vi "SCCSup Build Backend VI Path.vi"(6 "scc operation":T1, 9 "provider location":string, 11 "caller path":path) -> (2 "scc backend VI path":path)   [LabVIEW 2020]
uses:
  <vilib>/SourceControl/sccapi/SCCAPI SCC Operations.ctl
  <vilib>/SourceControl/sccapi/NI_SCC.lvlib
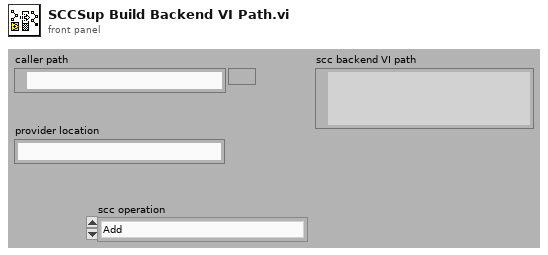
[diagram p1: front panel]
types:
  T1 = typedef "NI_SCC.lvlib/SCCAPI SCC Operations.ctl" = enum16{"Add", "Check In", "Check Out", "Close Project", "Compare Files", "Compare VIs", "Configure Project", "File History", "File Properties", "File Status", "Find All Providers", "Get Advanced Command Options", "Get File Copy", "Get Latest Version", "Get Project Name", "Get StaticVI Path", "Initialize", "Not A Source Control Reference", "Open Project", "Provider Supports Functionality", "Remove", "Run Provider", "Undo Check Out", "Uninitialize", "Is File In Local Path"}
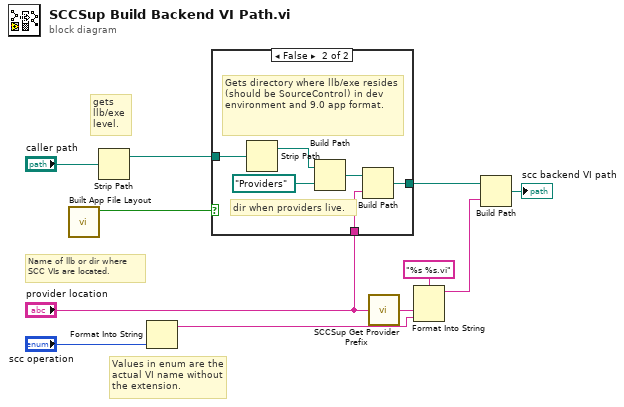
[diagram p0: block diagram]
diagram:
  # "Values in enum are the actual VI name without the extension."
  # "Name of llb or dir where SCC VIs are located."
  # "gets llb/exe level."
  n1 = call <vilib>:"Built App File Layout.vi"() -> ("Legacy Layout?"=w1:bool)  [unwired: 1 in, 10 out]
  n2 = Strip Path(path="caller path") -> (stripped path=w2:path)  [unwired: 1 out]
  n3 = Format Into String("scc operation") -> (resulting string=w3:string)  [unwired: 3 in, 1 out]
  n4 = case shown="False" w1 {
    tunnel: "provider location" -> [_ w18]
    tunnel: w2 -> [w12 w14]
    tunnel: [w12 w16] -> w7
    frame True {
      # "All files are at the same level in an exe, so there is no need to build up a directory heirarchy."
    }
    frame False {
      # "dir when providers live."
      # "Gets directory where llb/exe resides (should be SourceControl) in dev environment and 9.0 app format."
      n5 = Strip Path(path=w14) -> (stripped path=w13:path)  [unwired: 1 out]
      n6 = Build Path(base path=w13, name or relative path=path "Providers") -> (appended path=w17:path)
      n7 = Build Path(base path=w17, name or relative path=w18) -> (appended path=w16:path)
    }
  }
  n8 = call <vilib>:"SCCSup Get Provider Prefix.vi"("location"="provider location") -> ("prefix"=w10:string)  [unwired: 6 out]
  n9 = Format Into String(format string="%s %s.vi" ("Format String"), w10, w3) -> (resulting string=w6:string)  [unwired: 2 in, 1 out]
  n10 = Build Path(base path=w7, name or relative path=w6) -> (appended path=→"scc backend VI path":path)
